vi "MC - Test Message String.vi"(0 "message string":string) -> (1 "valid message":bool, 2 "message string is \"message\"":bool)   [LabVIEW 2015]
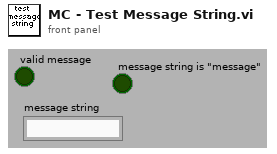
[diagram p1: front panel]
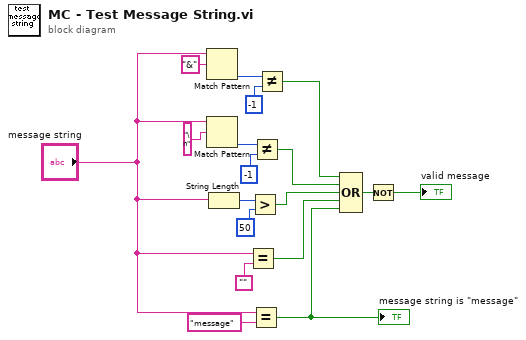
[diagram p0: block diagram]
diagram:
  n1 = Match Pattern(string="message string", regular expression="&") -> (offset past match=w9:i32)  [unwired: 4 out]
  n2 = Match Pattern(string="message string", regular expression="\n") -> (offset past match=w14:i32)  [unwired: 4 out]
  n3 = String Length(string="message string") -> (length=w17:i32)
  n4 = Equal?(x="message string", y="") -> (x = y?=w6:bool)
  n5 = Greater?(x=w17, y=50) -> (0:w11:bool)
  n6 = Equal?(x="message string", y="message") -> (x = y?=w1:bool)
  "message string is \"message\"" <- w1
  n7 = Not Equal?(x=w14, y=-1) -> (x != y?=w12:bool)
  n8 = Not Equal?(x=w9, y=-1) -> (x != y?=w7:bool)
  n9 = Compound Arithmetic op=OR(w7, w12, w11, w6, w1) -> (w5:bool)
  n10 = Not(x=w5) -> (.not. x?=→"valid message":bool)
